vi "Cross Baseline.vi"(3 "error in":errorcluster) -> (10 "error out":errorcluster)   [LabVIEW 2016]
uses:
  Refname/Motors.ctl
  Refname/Refname to String (Motors).vi
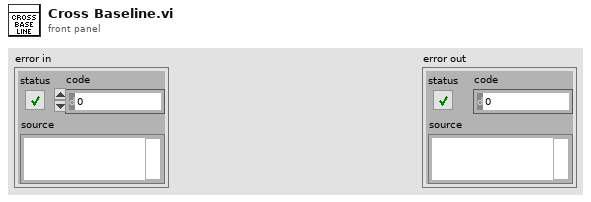
[diagram p1: front panel]
types:
  T1 = typedef "Motors.ctl" = enum16{"Wheel 1", "Swerve 1", "Wheel 2", "Swerve 2", "Wheel 3", "Swerve 3", "Wheel 4", "Swerve 4"}
  T2 = typedef "WPI_MotorControlDeviceRef.ctl" = cluster{"DeviceStatus":errorcluster, "Type":T3, "PWM":cluster{"PWM Channel":T4, "DeadBand":T5}, "CAN":cluster{"Device Number":u8, "SetOutput VI Ref":variant, "GetOutput VI Ref":variant, "Enable VI Ref":variant, "Disable VI Ref":variant, "Data":variant}, "Invert":bool}
  T3 = typedef "WPI_MotorControlType.ctl" = enum16{"PWM", "CAN"}
  T4 = typedef "FPGA_DIOPWMChannel.ctl" = enum8{"PWM 0", "PWM 1", "PWM 2", "PWM 3", "PWM 4", "PWM 5", "PWM 6", "PWM 7", "PWM 8", "PWM 9", "PWM MXP 0", "PWM MXP 1", "PWM MXP 2", "PWM MXP 3", "PWM MXP 4", "PWM MXP 5", "PWM MXP 6", "PWM MXP 7", "PWM MXP 8", "PWM MXP 9", "Invalid"}
  T5 = typedef "WPI_PWMDeadband.ctl" = cluster{"Name":string, "maxPositivePwm":i32, "minPositivePwm":i32, "centerPwm":i32, "maxNegativePwm":i32, "minNegativePwm":i32, "angularRange":u16}
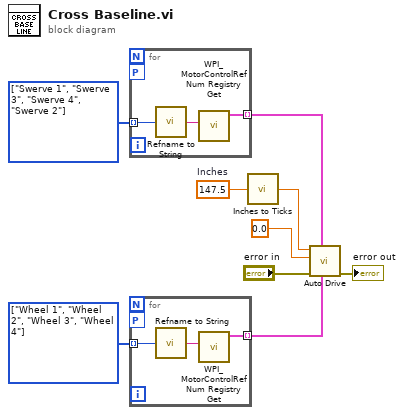
[diagram p0: block diagram]
diagram:
  w3 = T1[] [enum."Wheel 1", enum."Wheel 2", enum."Wheel 3", enum."Wheel 4"] items=["Wheel 1", "Swerve 1", "Wheel 2", "Swerve 2", "Wheel 3", "Swerve 3", "Wheel 4", "Swerve 4"]
  w4 = T1[] [enum."Swerve 1", enum."Swerve 3", enum."Swerve 4", enum."Swerve 2"] items=["Wheel 1", "Swerve 1", "Wheel 2", "Swerve 2", "Wheel 3", "Swerve 3", "Wheel 4", "Swerve 4"]
  w7 = 147.5  # Inches
  n1 = for {
    workers-P: _ -> [_]
    tunnel: w4 -> [w12] mode=indexing
    tunnel: [w10] -> w1 mode=indexing
    n2 = call-poly "Refname to String.vi"("Enum"=w12) -> ("String"=w11:string)
    n3 = call <vilib>:"WPI_MotorControlRefNum Registry Get.vi"("refnum name"=w11) -> ("MotorControlDevRef"=w10:T2)  [unwired: 9 in, 1 out]
  }
  n4 = for {
    workers-P: _ -> [_]
    tunnel: w3 -> [w15] mode=indexing
    tunnel: [w13] -> w2 mode=indexing
    n5 = call-poly "Refname to String.vi"("Enum"=w15) -> ("String"=w14:string)
    n6 = call <vilib>:"WPI_MotorControlRefNum Registry Get.vi"("refnum name"=w14) -> ("MotorControlDevRef"=w13:T2)  [unwired: 9 in, 1 out]
  }
  n7 = call "Inches to Ticks.vi"("Inches"=w7) -> ("Ticks"=w8:dbl)
  n8 = call "Auto Drive.vi"("Wheel DevRef"=w2, "Swerve DevRef"=w1, "error in"="error in", "Drive Angle"=0.0, "Ticks(Distance)"=w8) -> ("error out"=→"error out":errorcluster)  [unwired: 6 in]
